vi "Carbide-Get-ActualStateName.vi"(8 "Error In":errorcluster) -> (0 "Error Out":errorcluster, 3 "body":string)   [LabVIEW 2014]
doc: "André Romero - 2021\nandretec@ifsc.usp.br\nIFSC - USP"
uses:
  Carbide-Global.vi
  <vilib>/httpClient/LabVIEWHTTPClient.lvlib
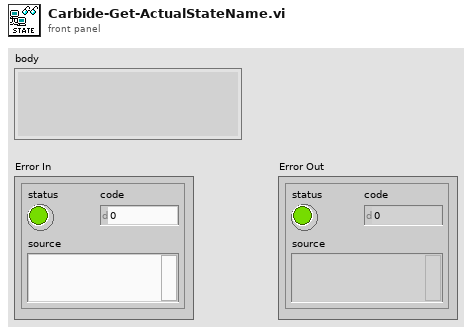
[diagram p1: front panel]
types:
  T1 = typedef "LabVIEWHTTPClient.lvlib/ClientHandle.ctl" = refnum<k1>
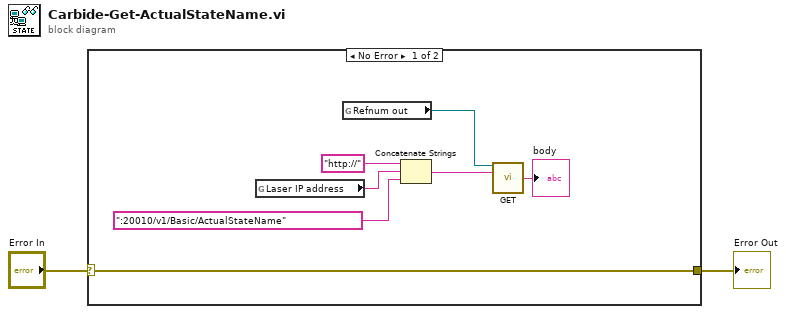
[diagram p0: block diagram]
diagram:
  n1 = case shown="No Error" "Error In" {
    selector: "Error In" -> [w4 w10]
    tunnel: [w4 w10] -> w1
    frame No Error {
      n2 = global read "Carbide-Global.vi" "Laser IP address"() -> (w6:string)
      n3 = global read "Carbide-Global.vi" "Refnum out"() -> (w9:T1)
      n4 = Concatenate Strings("http://" ("string"), w6, ":20010/v1/Basic/ActualStateName" ("string")) -> (w8:string)
      n5 = call <vilib>:"GET.vi"("client handle"=w9, "url"=w8) -> ("body"=→"body":string)  [unwired: 10 in, 3 out]
    }
    frame Error {
    }
  }
  "Error Out" <- w1
